vi "Bin Periodic Waveform.vi"(9 "Bin size":dbl=0.05, 10 "Y Array":dbl[](array[numeric]), 11 "X Array":dbl[](array[numeric])) -> ()   [LabVIEW 2016]
uses:
  Bin Average/Bin Average.lvclass
panel:
  out "XY Graph":cluster{"Array":dbl[], "Array":dbl[]}[](graph)
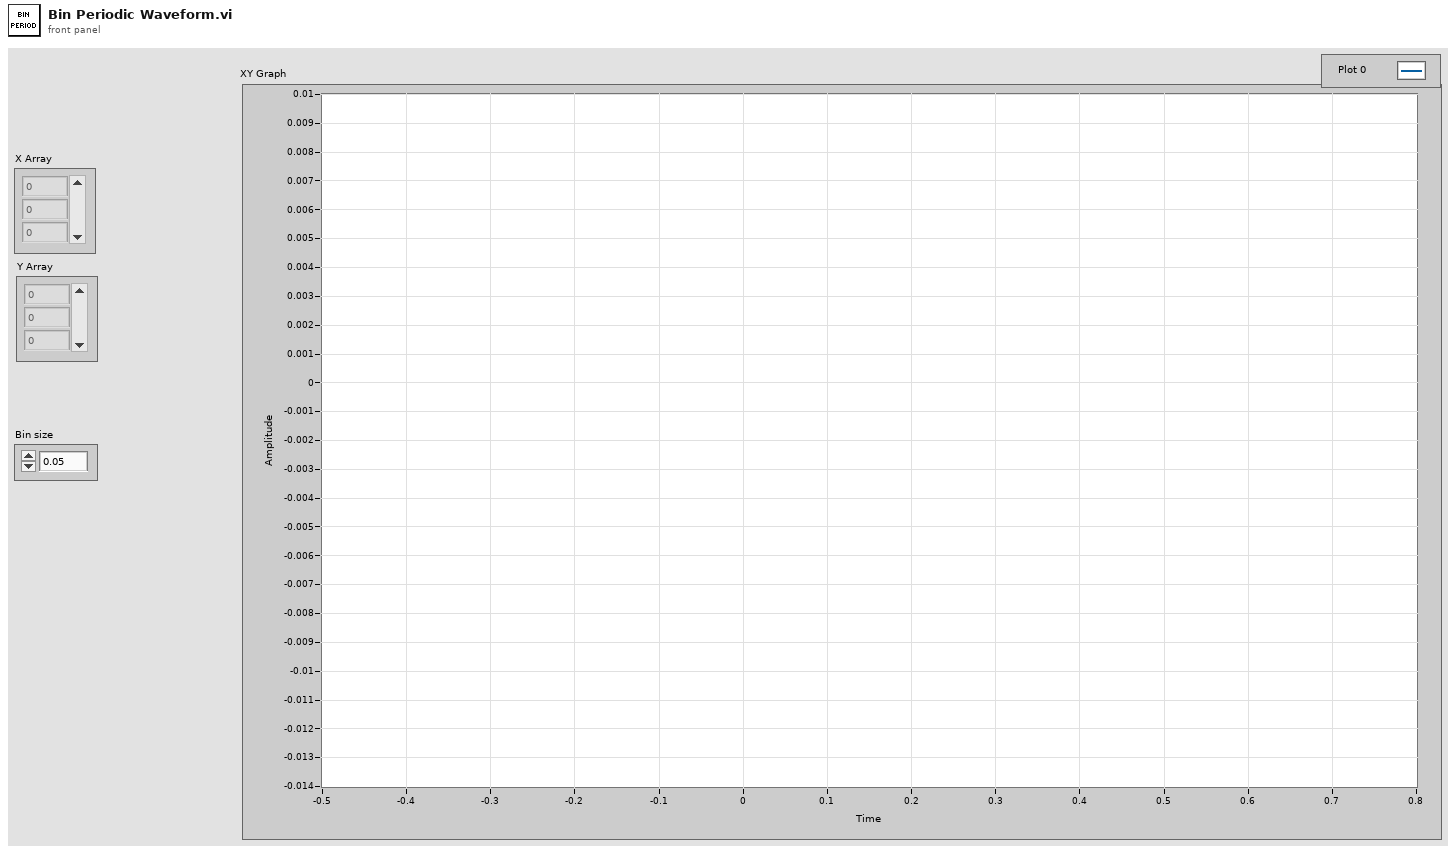
[diagram p1: front panel]
types:
  T1 = cluster{"X ref array":dbl[], "Binned average":dbl[]}
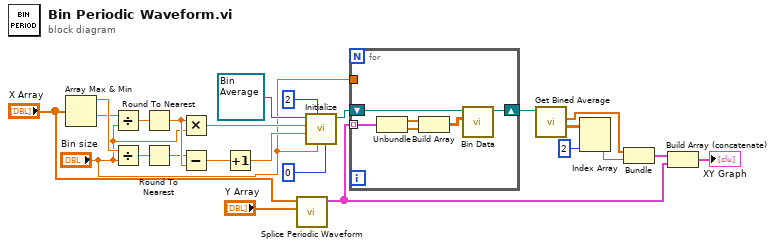
[diagram p0: block diagram]
diagram:
  n1 = Array Max & Min(array="X Array") -> (max value=w18:dbl, min value=w17:dbl)  [unwired: 2 out]
  n2 = Divide(x=w17, y="Bin size") -> (x/y=w20:dbl)
  n3 = Divide(x=w18, y="Bin size") -> (x/y=w19:dbl)
  n4 = Round To Nearest(number=w20) -> (nearest integer value=w22:dbl)
  n5 = Round To Nearest(number=w19) -> (nearest integer value=w21:dbl)
  n6 = Multiply(x=w22, y="Bin size") -> (x*y=w15:dbl)
  n7 = Subtract(x=w21, y=w22) -> (x-y=w14:dbl)
  n8 = Increment(x=w14) -> (x+1=w13:dbl)
  n9 = call "Splice Periodic Waveform.vi"("Y Array"="Y Array", "X Array"="X Array") -> ("Output arrays"=w4:cluster{"Array":dbl[], "Array":dbl[]}[])  [unwired: 8 in, 1 out]
  n10 = call-dynamic "Initialize.vi"("X column"=0, "Bin"="Bin size", "Number of columns"=2, "Number of rows"=w13, "Start"=w15, "Bin Average in"=refnum<class "Bin Average.lvclass"> refnum ("Bin Average.lvclass")) -> ("Bin Average out"=w9:refnum<class "Bin Average.lvclass">)  [unwired: 4 in, 1 out]
  n11 = for {
    tunnel: w4 -> [w30] mode=indexing
    tunnel: "Bin size" -> [_]
    shift-right: [w25] -> w8
    shift-left: w9 -> [w27]
    n12 = Unbundle(w30) -> ("Array"=w29:dbl[], "Array"=w28:dbl[])
    n13 = Build Array(w29, w28) -> (w26:dbl[][])
    n14 = call-dynamic "Bin Data.vi"("Data in"=w26, "Bin Average in"=w27) -> ("Bin Average out"=w25:refnum<class "Bin Average.lvclass">)  [unwired: 8 in, 1 out]
  }
  n15 = call-dynamic "Get Bined Average.vi"("Bin Average in"=w8) -> ("Binned average"=w7:dbl[][], "X ref array"=w6:dbl[])  [unwired: 7 in, 2 out]
  n16 = Index Array(array=w7, index (col)=2 ("disabled index (col)")) -> (element=w2:dbl[])  [unwired: 1 in]
  n17 = Bundle("X ref array"=w6, "Binned average"=w2) -> (w5:T1)  [unwired: 1 in]
  n18 = Build Array (concatenate)(w5, w4) -> (→"XY Graph":cluster{"Array":dbl[], "Array":dbl[]}[])
